vi "Control Relay.vi"   [LabVIEW 2019, in "Relay-Box.lvclass"]
uses:
  Relay-Box.lvclass
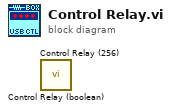
[diagram p0: block diagram]
diagram:
  n1 = call "Control Relay (boolean).vi"() -> ()  [unwired: 11 in, 1 out]
  n2 = call "Control Relay (256).vi"() -> ()  [unwired: 11 in, 1 out]
